vi "FPGA_Main.vi"() -> ()   [LabVIEW 2013]
uses:
  Battery/TypeDefs/SPI_State.ctl
  <vilib>/Platform/TimedLoop/XDataNode/timing_clust.ctl
  <vilib>/Platform/TimedLoop/XDataNode/nitl_modes.ctl
  <vilib>/Platform/TimedLoop/XDataNode/wakeup.ctl
  <vilib>/rvi/Emulation/niFpgaSctlEmulationGetInTimedLoop.vi
  <vilib>/rvi/Emulation/niFpgaEmulationReportErrorSimple.vi
  <vilib>/rvi/Emulation/niFpgaGetClockAttributes.vi
  <vilib>/rvi/Emulation/niFpgaCriticalErrorInLSC.vi
  <vilib>/rvi/eio/common/nirviEmuTemplateMethod_errors.vi
  <vilib>/Platform/TimedLoop/XDataNode/XDataNode.xnode
  <vilib>/eio/EIONode/EIONode.xnode
  <vilib>/rvi/Analysis/measure/butterworth/XNode/niFpgaButterworthFilter.xnode
  <vilib>/Platform/TimedLoop/XDataNode/XDNodeRunTimeDep.lvlib
  <vilib>/robotics/utilities/FPGA Utilities/NI_Robotics_FPGA Utilities.lvlib
  <vilib>/robotics/Utilities/FPGA Utilities/Generate Digital Pulse (uSec).vi
panel:
  out "Unfiltered Battery Voltage ADC Output":u16
  in  "Winch Duty (uSec)":u32
  in  "Rudder Duty (uSec)":u32
  out "Filtered Battery Voltage ADC Output":u32
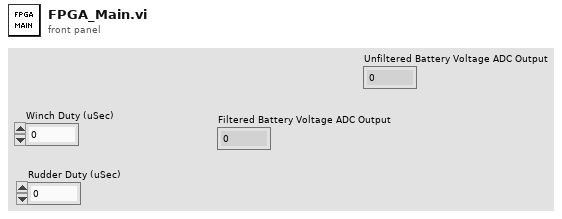
[diagram p1: front panel]
types:
  T1 = typedef "SPI_State.ctl" = enum8{"Start Read", "Transition", "Wait Cycles", "End Read"}
  T2 = typedef "XDNodeRunTimeDep.lvlib/timing_clust.ctl" = cluster{"Expected End [f-1]":u64, "Actual End [f-1]":u64, "Finished Late? [f-1]":bool, "Expected End [i-1]":u64, "Actual End [i-1]":u64, "Finished Late? [i-1]":bool, "Expected Start [i]":u64, "Actual Start [i]":u64, "Expected Start [f]":u64, "Actual Start [f]":u64, "Source Name":string, "Structure Name":string, "Period":i64, "Deadline":i64, "Offset":i64, "Start":i64, "Priority":i32, "Timeout":i32, "Mode":T3, "Wakeup Reason":T4, "Error":errorcluster, "Source Type":string, "Secondary Source Type":string, "Global End Time":u64, "Global Start Time":u64, "Frame Duration":u64, "Iteration Duration":u64, "Assigned CPU":i32, "I/O Scan Engine Mode":u32}
  T3 = typedef "XDNodeRunTimeDep.lvlib/nitl_modes.ctl" = enum32{"No Change", "Process missed periods, maintain original phase", "Discard missed periods, maintain original phase", "Process missed periods, ignore original phase", "Discard missed periods, ignore original phase"}
  T4 = typedef "XDNodeRunTimeDep.lvlib/wakeup.ctl" = enum32{"Normal", "Aborted", "Asynchronous wakeup", "Timing source error", "Timed loop error", "Timeout"}
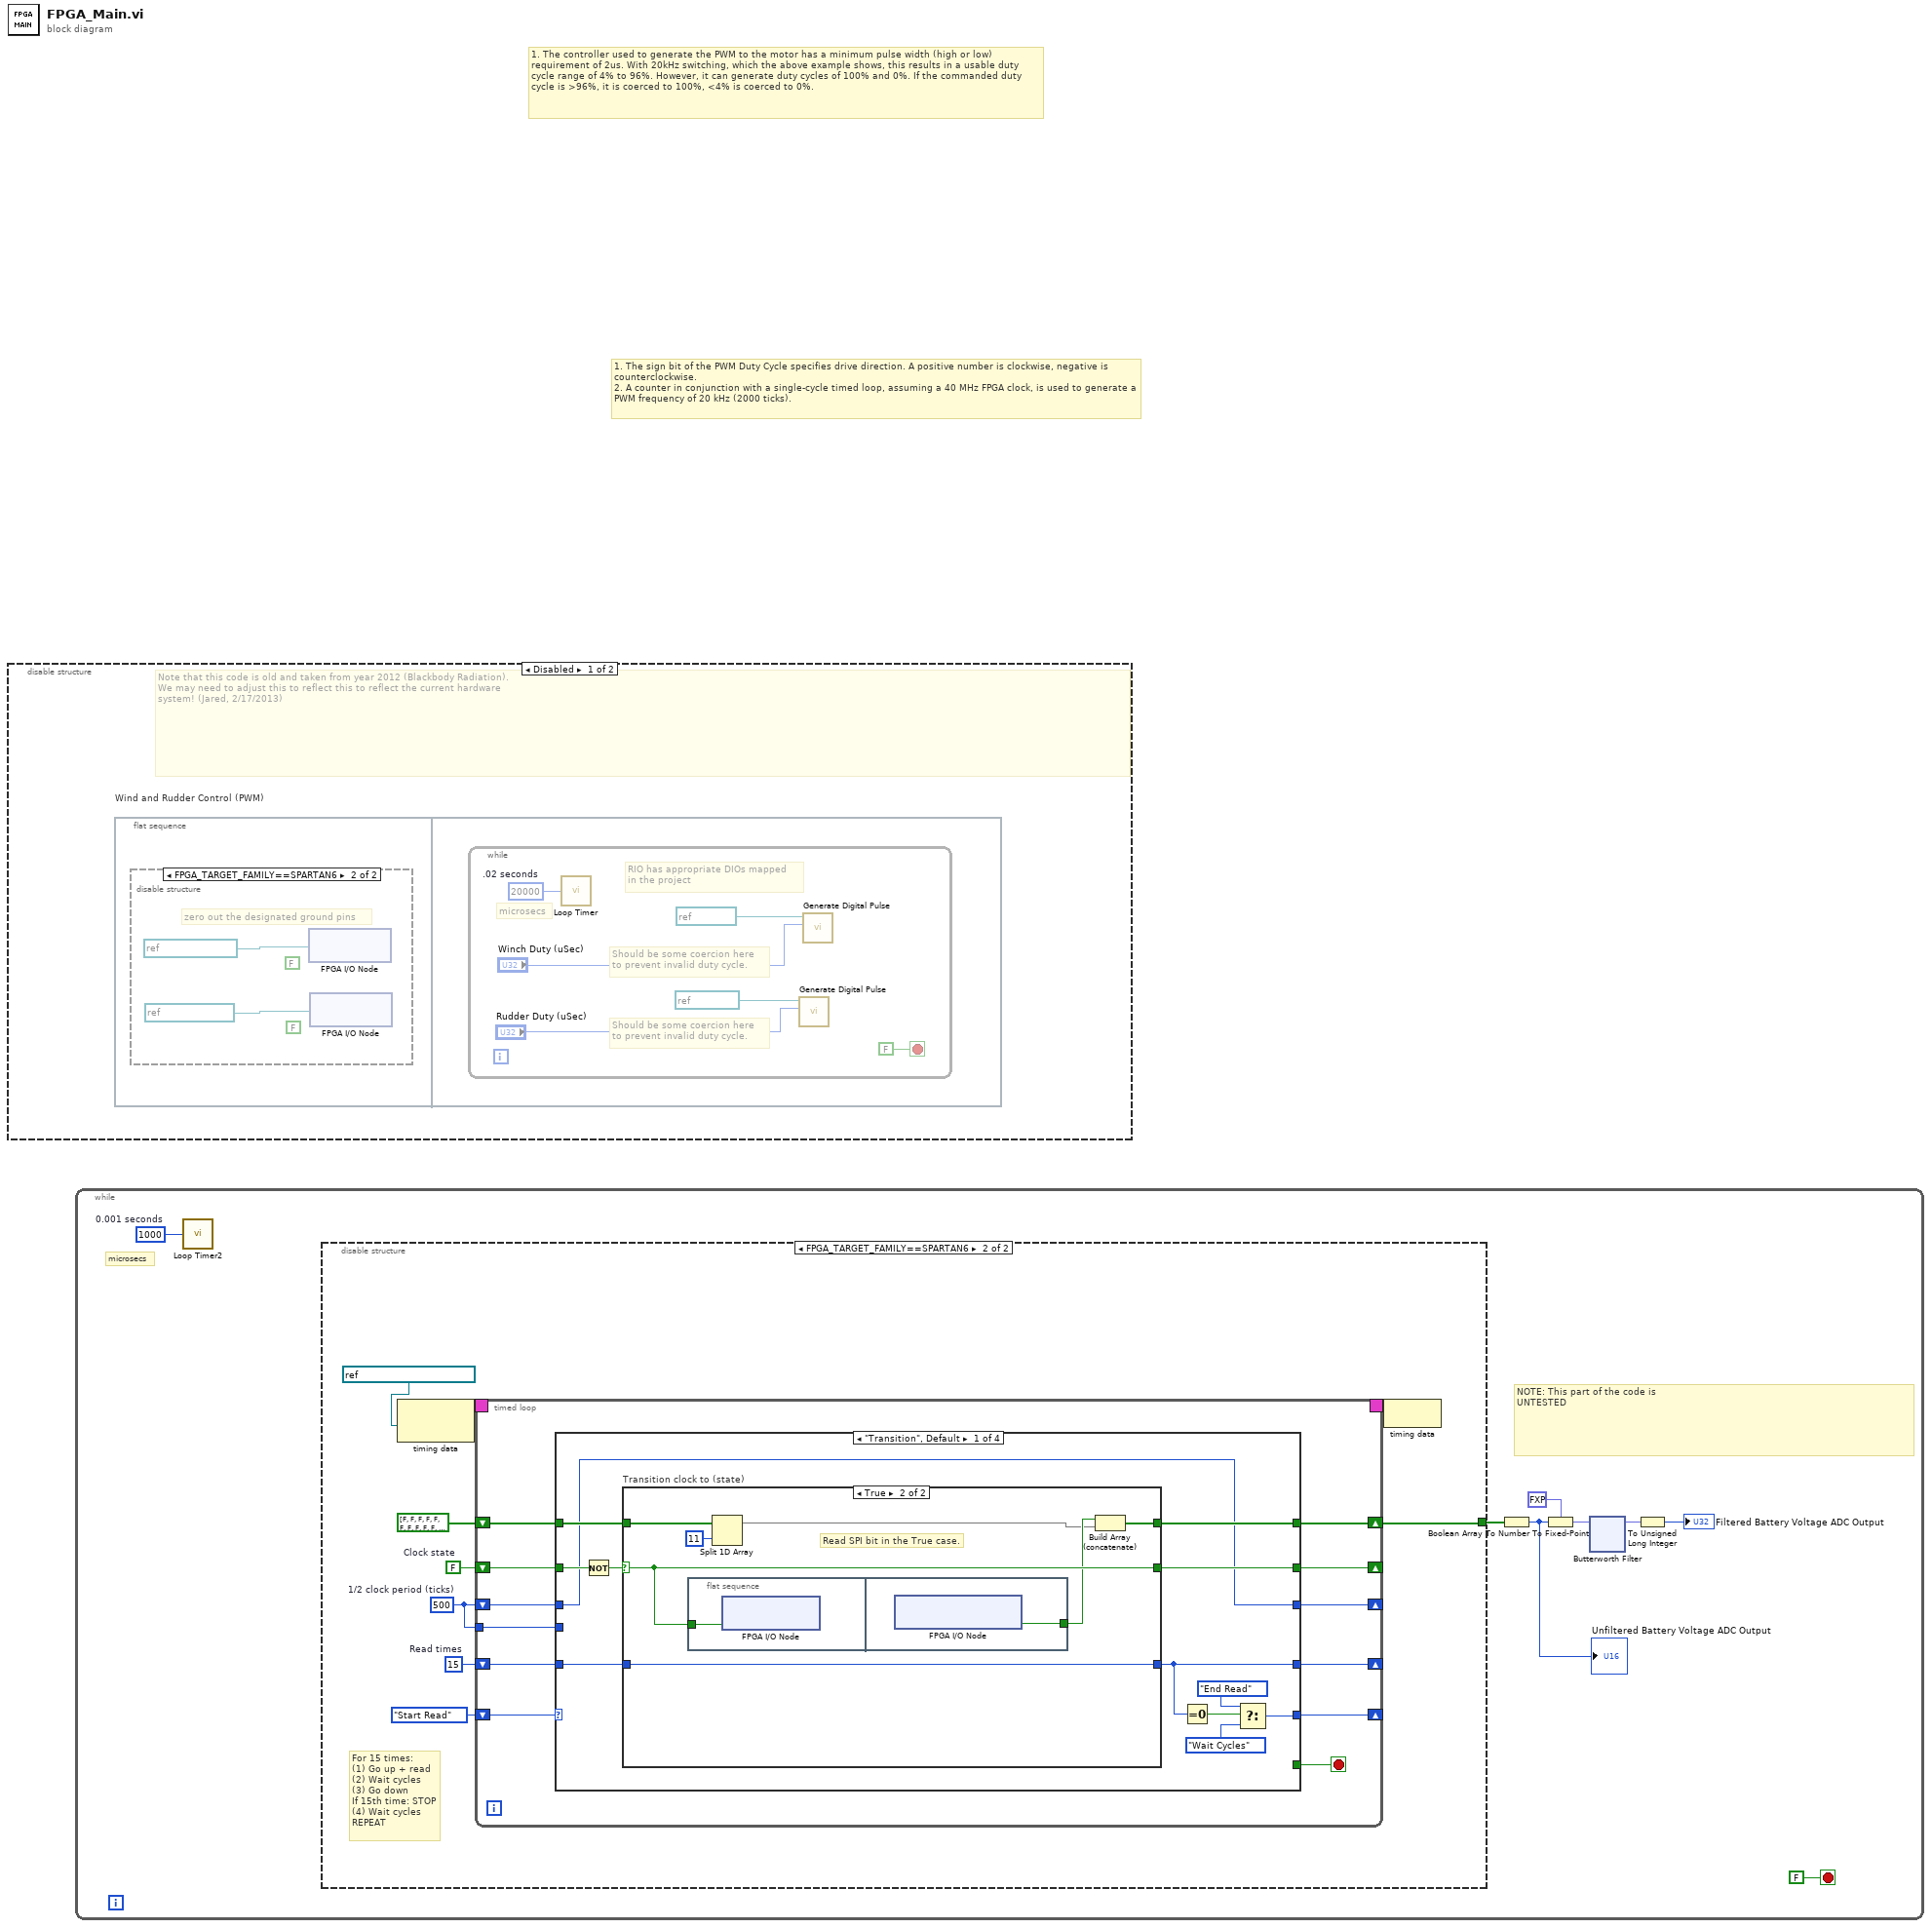
[diagram p0: block diagram]
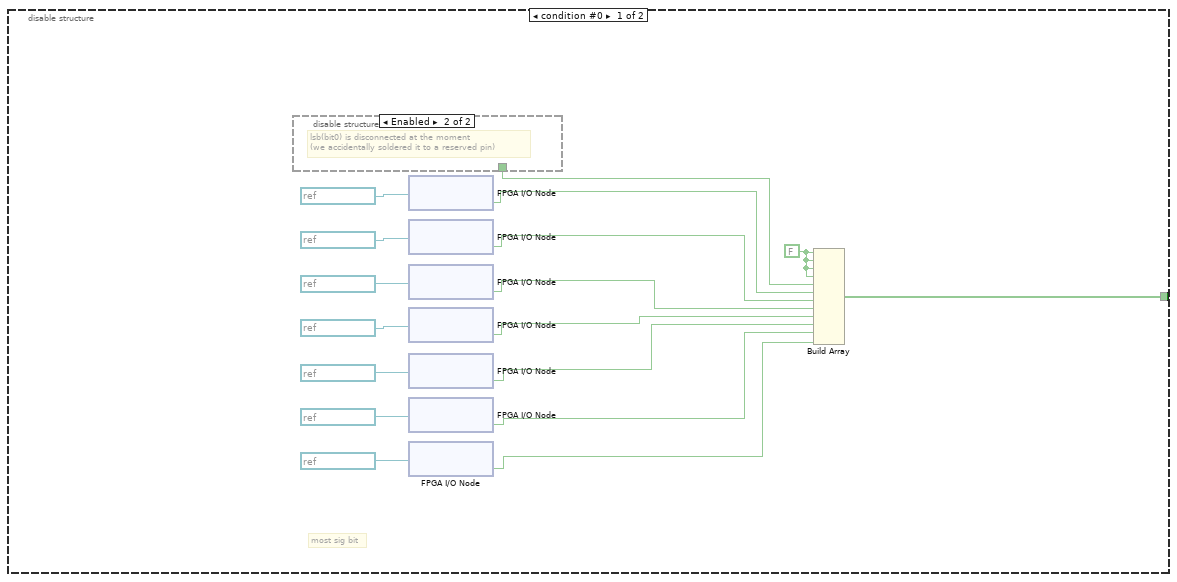
[diagram p4: hidden frame]
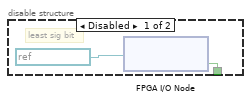
[diagram p5: hidden frame]
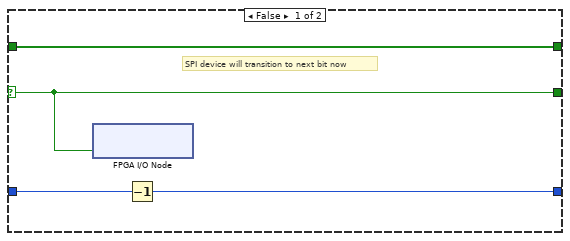
[diagram p6: hidden frame]
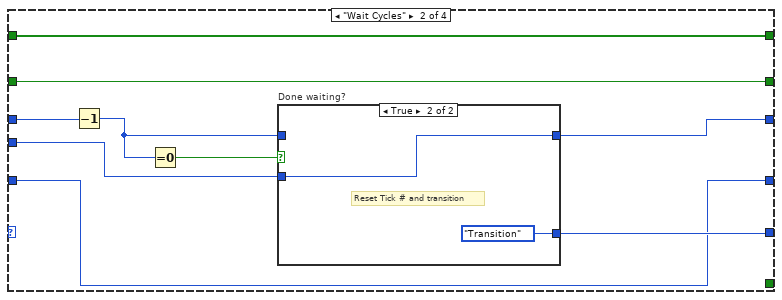
[diagram p7: hidden frame]
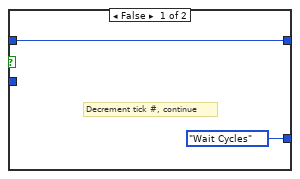
[diagram p8: hidden frame]
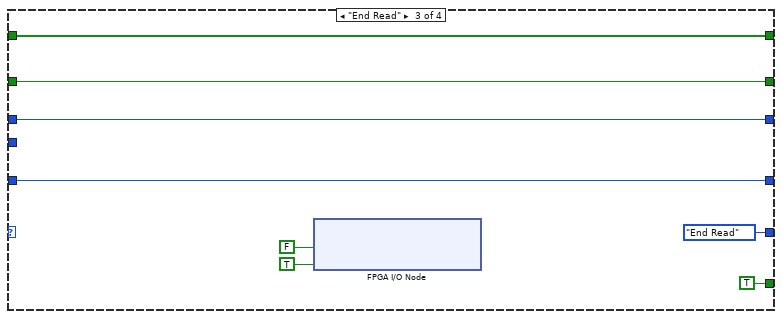
[diagram p9: hidden frame]
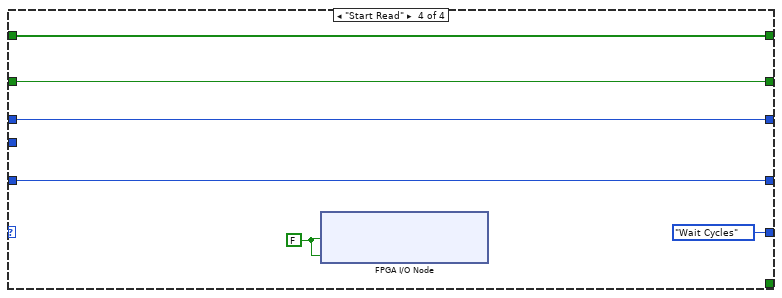
[diagram p10: hidden frame]
diagram:
  # "1. The sign bit of the PWM Duty Cycle specifies drive direction. A positive number is clockwise, negative is counterclockwise.\n2. A counter in conjunction with a single-cycle timed loop, assuming a 40 MHz FPGA clock, is used to generate a PWM frequency of 20 kHz (2000 ticks)."
  # "1. The controller used to generate the PWM to the motor has a minimum pulse width (high or low) requirement of 2us. With 20kHz switching, which the above example shows, this results in a usable duty cycle range of 4% to 96%. However, it can generate duty cycles of 100% and 0%. If the commanded duty cycle is >96%, it is coerced to 100%, <4% is coerced to 0%."
  n1 = disable-structure shown="Disabled" {
    frame Disabled {
      # "Note that this code is old and taken from year 2012 (Blackbody Radiation).\nWe may need to adjust this to reflect this to reflect the current hardware\nsystem! (Jared, 2/17/2013)"
      n2 = flat-sequence "Wind and Rudder Control (PWM)" {
        frame #0 {
          n3 = disable-structure shown="FPGA_TARGET_FAMILY==SPARTAN6" {
            frame condition #0 {
            }
            frame condition #1 (active) {
              w3 = FALSE ("I/O Item")
              w4 = FALSE ("I/O Item")
              # "zero out the designated ground pins"
              n4 = xnode "FPGA I/O Node"("FPGA I/O In"=refnum<k21> "Rudder_GND" ("FPGA digital output")) -> ()  [unwired: 1 in, 1 out]
              n5 = xnode "FPGA I/O Node"("FPGA I/O In"=refnum<k21> "Winch_GND" ("FPGA digital output")) -> ()  [unwired: 1 in, 1 out]
            }
          }
        }
        frame #1 {
          n6 = while {
            stop <- FALSE stop-if-true
            w10 = u32 20000  # .02 seconds
            # "microsecs"
            # "Should be some coercion here\nto prevent invalid duty cycle."
            # "Should be some coercion here\nto prevent invalid duty cycle."
            # "RIO has appropriate DIOs mapped\nin the project"
            n7 = call "Loop Timer"("Count(uSec)"=w10) -> ()  [unwired: 1 out]
            n8 = call-poly <vilib>:"Generate Digital Pulse.vi"("pulse width (uSec)"="Rudder Duty (uSec)", "FPGA digital output"=refnum<k21> "Rudder") -> ()  [unwired: 10 in]
            n9 = call-poly <vilib>:"Generate Digital Pulse.vi"("pulse width (uSec)"="Winch Duty (uSec)", "FPGA digital output"=refnum<k21> "Winch") -> ()  [unwired: 10 in]
          }
        }
      }
    }
    frame Enabled {
    }
  }
  n10 = while {
    stop <- FALSE stop-if-true
    w11 = u32 1000  # 0.001 seconds
    # "microsecs"
    # "NOTE: This part of the code is\nUNTESTED"
    n11 = call "Loop Timer2"("Count(uSec)"=w11) -> ()  [unwired: 1 out]
    n12 = disable-structure shown="FPGA_TARGET_FAMILY==SPARTAN6" {
      disable-tunnel: [w27 w48] -> w18
      frame condition #0 {
        w26 = FALSE ("element")
        # "most sig bit"
        n13 = disable-structure shown="Enabled" {
          disable-tunnel: [w43 _] -> w28
          frame Disabled {
            # "least sig bit"
            n14 = xnode "FPGA I/O Node"("FPGA I/O In"=refnum<k21> "VBatt bit0") -> ("I/O Item"=w43:bool)  [unwired: 1 out]
          }
          frame Enabled {
            # "lsb(bit0) is disconnected at the moment\n(we accidentally soldered it to a reserved pin)"
          }
        }
        n15 = xnode "FPGA I/O Node"("FPGA I/O In"=refnum<k21> "VBatt bit1") -> ("I/O Item"=w36:bool)  [unwired: 1 out]
        n16 = xnode "FPGA I/O Node"("FPGA I/O In"=refnum<k21> "VBatt bit2") -> ("I/O Item"=w37:bool)  [unwired: 1 out]
        n17 = xnode "FPGA I/O Node"("FPGA I/O In"=refnum<k21> "VBatt bit3") -> ("I/O Item"=w38:bool)  [unwired: 1 out]
        n18 = xnode "FPGA I/O Node"("FPGA I/O In"=refnum<k21> "VBatt bit4") -> ("I/O Item"=w39:bool)  [unwired: 1 out]
        n19 = xnode "FPGA I/O Node"("FPGA I/O In"=refnum<k21> "VBatt bit5") -> ("I/O Item"=w40:bool)  [unwired: 1 out]
        n20 = xnode "FPGA I/O Node"("FPGA I/O In"=refnum<k21> "VBatt bit6") -> ("I/O Item"=w41:bool)  [unwired: 1 out]
        n21 = xnode "FPGA I/O Node"("FPGA I/O In"=refnum<k21> "VBatt bit7") -> ("I/O Item"=w42:bool)  [unwired: 1 out]
        n22 = Build Array(w26, w26, w26, w26, w28, w36, w37, w38, w39, w40, w41, w42) -> (w27:bool[])
      }
      frame condition #1 (active) {
        w49 = u32 500  # 1/2 clock period (ticks)
        w50 = FALSE  # Clock state
        w51 = u8 15  # Read times
        # "For 15 times:\n(1) Go up + read\n(2) Wait cycles\n(3) Go down\nIf 15th time: STOP\n(4) Wait cycles\nREPEAT"
        n23 = node-c288(refnum<k21> "40 MHz Onboard Clock" ("Source Name")) -> (w47:T2)
        n24 = timed-loop {
          shift-right: [w58] -> _
          shift-left: SPI_State."Start Read" ("Action") -> [w65]
          shift-right: [w61] -> w48
          shift-left: bool[] [FALSE, FALSE, FALSE, FALSE, FALSE, FALSE, FALSE, FALSE, FALSE, FALSE, FALSE, FALSE] ("Battery Voltage") -> [w62]
          shift-right: [w63] -> _
          shift-left: w50 -> [w64]
          tunnel: w49 -> [w56]
          shift-right: [w55] -> _
          shift-left: w49 -> [w57]
          shift-right: [w59] -> _
          shift-left: w51 -> [w60]
          timing: w47 -> [_]
          timing-out: [_] -> w46
          stop <- w54 stop-if-true
          n25 = case shown="\"Transition\", Default" w65 {
            tunnel: w64 -> [w77 w99 w107 w115]
            tunnel: [w76 w99 w107 w115] -> w63
            tunnel: w62 -> [w74 w98 w106 w116]
            tunnel: [w73 w98 w106 w116] -> w61
            tunnel: w60 -> [w72 w91 w110 w113]
            tunnel: [w70 w91 w110 w113] -> w59
            tunnel: [w68 w94 SPI_State."End Read" ("Action") SPI_State."Wait Cycles" ("Action")] -> w58
            tunnel: w57 -> [w71 w97 w108 w114]
            tunnel: w56 -> [_ w92 _ _]
            tunnel: [w71 w93 w108 w114] -> w55
            tunnel: [_ _ TRUE _] -> w54
            frame "Transition", Default {
              n26 = Not(x=w77) -> (.not. x?=w75:bool)
              n27 = case "Transition clock to (state)" shown="True" w75 {
                selector: w75 -> [w81 w88]
                tunnel: [w81 w88] -> w76
                tunnel: w74 -> [w78 w84]
                tunnel: [w78 w82] -> w73
                tunnel: w72 -> [w80 w86]
                tunnel: [w79 w86] -> w70
                frame False {
                  # "SPI device will transition to next bit now"
                  n28 = xnode "FPGA I/O Node"("VBatt_Clock"=w81) -> ()  [unwired: 1 in, 1 out]
                  n29 = Decrement(x=w80) -> (x-1=w79:u8)
                }
                frame True {
                  # "Read SPI bit in the True case."
                  n30 = flat-sequence {
                    tunnel: w88 -> [w89]
                    tunnel: [w90] -> w85
                    frame #0 {
                      n31 = xnode "FPGA I/O Node"("VBatt_Clock"=w89) -> ()  [unwired: 1 in, 1 out]
                    }
                    frame #1 {
                      n32 = xnode "FPGA I/O Node"() -> ("VBatt_DigitalInput"=w90:bool)  [unwired: 1 in, 1 out]
                    }
                  }
                  n33 = Split 1D Array(array=w84, index=11) -> (first subarray=w83:bool[])  [unwired: 1 out]
                  n34 = Build Array (concatenate)(w85, w83) -> (w82:bool[])
                }
              }
              n35 = Equal To 0?(x=w70) -> (x = 0?=w69:bool)
              n36 = Select(t=SPI_State."End Read" ("Action"), s=w69, f=SPI_State."Wait Cycles" ("Action")) -> (s? t:f=w68:T1)
            }
            frame "Wait Cycles" {
              n37 = Decrement(x=w97) -> (x-1=w95:u32)
              n38 = Equal To 0?(x=w95) -> (x = 0?=w96:bool)
              n39 = case "Done waiting?" shown="True" w96 {
                tunnel: w95 -> [w100 _]
                tunnel: [SPI_State."Wait Cycles" ("Action") SPI_State."Transition" ("Action")] -> w94
                tunnel: [w100 w102] -> w93
                tunnel: w92 -> [_ w102]
                frame False {
                  # "Decrement tick #, continue"
                }
                frame True {
                  # "Reset Tick # and transition"
                }
              }
            }
            frame "End Read" {
              n40 = xnode "FPGA I/O Node"("VBatt_Clock"=FALSE ("VBatt_ChipSelectInverted"), "VBatt_ChipSelectInverted"=TRUE) -> ()  [unwired: 2 in, 2 out]
            }
            frame "Start Read" {
              w117 = FALSE ("VBatt_ChipSelectInverted")
              n41 = xnode "FPGA I/O Node"("VBatt_Clock"=w117, "VBatt_ChipSelectInverted"=w117) -> ()  [unwired: 2 in, 2 out]
            }
          }
        }
        n42 = node-c288(w46) -> ()
      }
    }
    n43 = Boolean Array To Number(Boolean array=w18) -> (number=w17:u16)
    "Unfiltered Battery Voltage ADC Output" <- w17
    n44 = To Fixed-Point(fixed-point type=fxp<+/-,32,33> 0.0 ("input data"), number=w17) -> (fixed-point=w15:fxp<+/-,32,33>)
    n45 = xnode "Butterworth Filter"("input data"=w15) -> ("output data"=w14:fxp<+/-,32,33>)  [unwired: 2 in]
    n46 = To Unsigned Long Integer(number=w14) -> (unsigned 32bit integer=→"Filtered Battery Voltage ADC Output":u32)
  }
